vi "TCP 기다림(SubVI).vi"(8 "error in":errorcluster caption="에러 입력(에러 없음)", 10 "기다림(ms)":u32, 11 "TCP 네트워크 연결 입력":refnum<k5>) -> (0 "error out":errorcluster caption="에러 출력", 3 "TCP 네트워크 연결 출력":refnum<k5>)   [LabVIEW 2014]
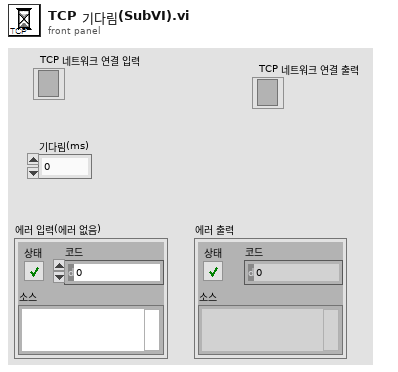
[diagram p1: front panel]
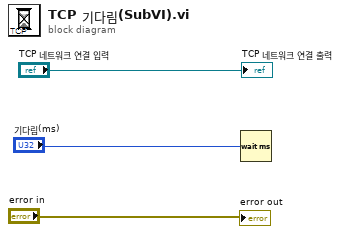
[diagram p0: block diagram]
diagram:
  n1 = Wait (ms)(milliseconds to wait="기다림(ms)") -> ()  [unwired: 1 out]
  "TCP 네트워크 연결 출력" <- "TCP 네트워크 연결 입력"
  "error out" <- "error in"
